vi "Is_TestDataInSpec- 单值-四舍五入.vi"(5 "数值":dbl format="%#_13g") -> (0 "进位舍位后值":dbl format="%#_13g", 1 "在规格内":bool)   [LabVIEW 2014]
uses:
  Controls/TestThreshold.ctl
panel:
  in  "量测内容":T1={"量测项目名称"="", "量测项阈值"={"下限"=0.0, "上限"=0.0}, "下限进位范围"=0.005, "上限舍位范围"=0.005, "修正系数k"=1.0, "补偿值b"=0.0, "单项测试数据个数"=1, "单位mm"=TRUE, "取消测试"=FALSE, "选择相机"=enum."相机1", "参与CPK计算量测项阈值"={"下限"=0.0, "上限"=0.0}} {"参与CPK计算量测项阈值"."上限" format="%#.4g"; "参与CPK计算量测项阈值"."下限" format="%#.4g"; "量测项阈值"."上限" format="%#.4g"; "量测项阈值"."下限" format="%#.4g"}
  # "~"
  # "~"
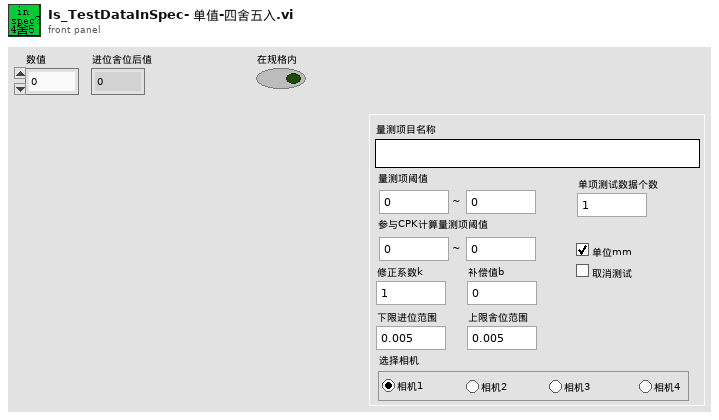
[diagram p1: front panel]
types:
  T1 = typedef "量测内容.ctl" = cluster{"量测项目名称":string, "量测项阈值":T2, "下限进位范围":dbl, "上限舍位范围":dbl, "修正系数k":dbl, "补偿值b":dbl, "单项测试数据个数":i32, "单位mm":bool, "取消测试":bool, "选择相机":enum32{"相机1", "相机2", "相机3", "相机4"}, "参与CPK计算量测项阈值":T2}
  T2 = typedef "TestThreshold.ctl" = cluster{"下限":dbl, "上限":dbl}
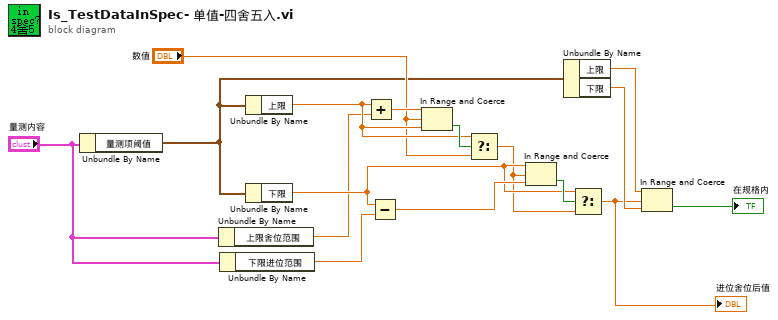
[diagram p0: block diagram]
diagram:
  n1 = Unbundle By Name("量测内容") -> ("量测项阈值"=w4:T2)
  n2 = Unbundle By Name("量测内容") -> ("上限舍位范围"=w2:dbl)
  n3 = Unbundle By Name("量测内容") -> ("下限进位范围"=w1:dbl)
  n4 = Unbundle By Name(w4) -> ("上限"=w14:dbl)
  n5 = Unbundle By Name(w4) -> ("下限"=w9:dbl)
  n6 = Add(x=w14, y=w2) -> (x+y=w16:dbl)
  n7 = Subtract(x=w9, y=w1) -> (x-y=w12:dbl)
  n8 = In Range and Coerce(upper limit=w16, x="数值", lower limit=w14) -> (In Range?=w15:bool)  [unwired: 1 out]
  n9 = Select(t=w14, s=w15, f="数值") -> (s? t:f=w8:dbl)
  n10 = In Range and Coerce(upper limit=w9, x=w8, lower limit=w12) -> (In Range?=w13:bool)  [unwired: 1 out]
  n11 = Unbundle By Name(w4) -> ("上限"=w10:dbl, "下限"=w11:dbl)
  n12 = Select(t=w9, s=w13, f=w8) -> (s? t:f=w6:dbl)
  "进位舍位后值" <- w6
  n13 = In Range and Coerce(upper limit=w10, x=w6, lower limit=w11) -> (In Range?=→"在规格内":bool)  [unwired: 1 out]
